vi "Waveform to XY (multiple).vi"(8 "error in (no error)":errorcluster, 11 "Waveform in":waveform(dbl)[](array[waveform])) -> (0 "error out":errorcluster, 3 "XY-data out":cluster{"X-array":dbl[], "Y-array":dbl[]}[](array[cluster]) {"Y-array" format="%.2p"; "X-array" format="%.2p"})   [LabVIEW 2019, in "xy_utilities.lvlib"]
doc: "Convert array of <b>Waveforms</b> to array of <b>XY-data<b>"
uses:
  xy_utilities.lvlib
  <vilib>/Waveform/WDTOps.llb/Waveform to XY Pairs.vi
  <vilib>/Waveform/WDTOps.llb/WDT Waveform to XY Pairs DBL.vi
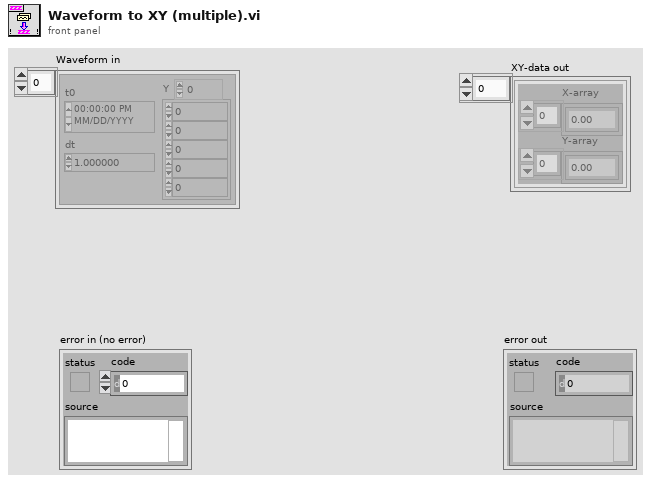
[diagram p1: front panel]
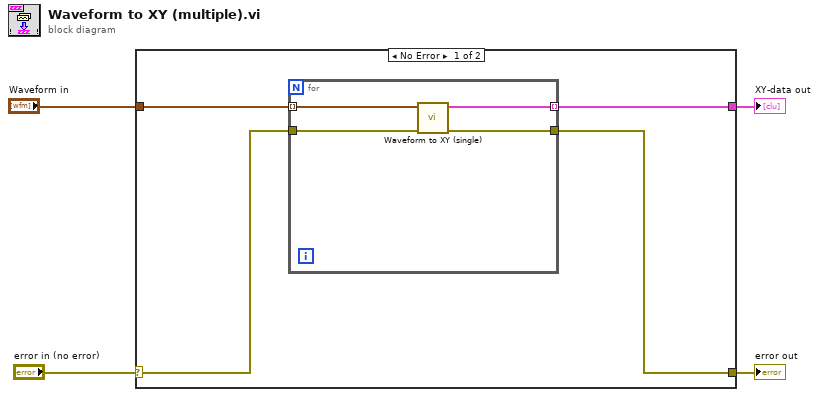
[diagram p0: block diagram]
diagram:
  n1 = case shown="No Error" "error in (no error)" {
    selector: "error in (no error)" -> [w7 w13]
    tunnel: [w5 w13] -> w3
    tunnel: "Waveform in" -> [w8 _]
    tunnel: [w6 _] -> w2
    frame No Error {
      n2 = for {
        tunnel: w8 -> [w12] mode=indexing
        tunnel: w7 -> [w11]
        tunnel: [w10] -> w5
        tunnel: [w9] -> w6 mode=indexing
        n3 = call "Waveform to XY (single).vi"("error in (no error)"=w11, "Waveform in"=w12) -> ("error out"=w10:errorcluster, "XY-data out"=w9:cluster{"X-array":dbl[], "Y-array":dbl[]})  [unwired: 8 in]
      }
    }
    frame Error {
    }
  }
  "error out" <- w3
  "XY-data out" <- w2
